vi "Shift Header to point to starting tag.vi"(6 "Byte stream offset\ninsertion point where \nnew data/tag added":u32, 7 "Litt/BigEnd":bool, 8 "error in":errorcluster, 9 "# bytes added\n(<0 means removed)":i32, 11 "Image Data":u8[](array[numeric])) -> (0 "error out":errorcluster, 1 "Shifted?":bool, 3 "Image Data Out":u8[](array[numeric]))   [LabVIEW 2013, in "Tiff reader.lvlib"]
doc: "This .vi shifts the data stream that is to be added into a stack so that the pointers now point to their new locations."
uses:
  Tiff reader.lvlib
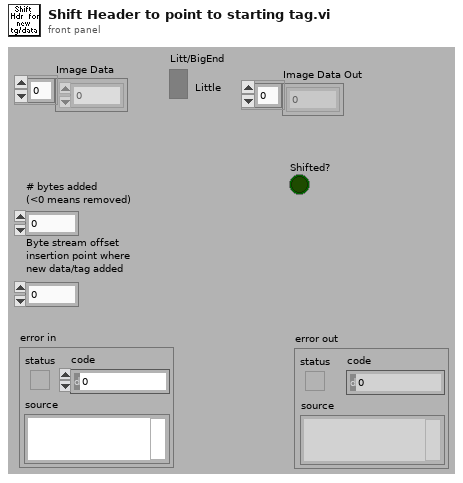
[diagram p1: front panel]
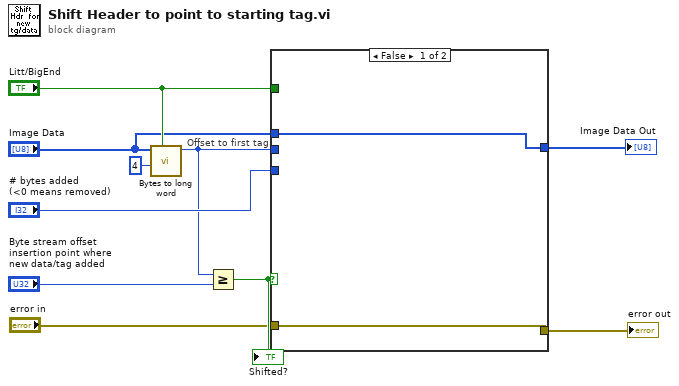
[diagram p0: block diagram]
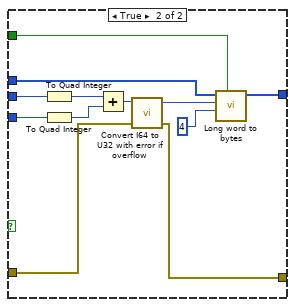
[diagram p2: hidden frame]
diagram:
  # "Offset to first tag"
  n1 = call "Bytes to long word.vi"("Litt/BigEnd"="Litt/BigEnd", "Index"=4, "Image Data in"="Image Data") -> ("U32"=w7:u32)  [unwired: 6 out]
  n2 = Greater Or Equal?(x=w7, y="Byte stream offset\ninsertion point where \nnew data/tag added") -> (x >= y?=w4:bool)
  "Shifted?" <- w4
  n3 = case shown="False" w4 {
    tunnel: "Image Data" -> [w12 w24]
    tunnel: [w12 w23] -> w6
    tunnel: w7 -> [_ w22]
    tunnel: "# bytes added\n(<0 means removed)" -> [_ w20]
    tunnel: "Litt/BigEnd" -> [_ w17]
    tunnel: "error in" -> [w11 w14]
    tunnel: [w11 w13] -> w2
    frame False {
    }
    frame True {
      n4 = To Quad Integer(1:w22) -> (0:w21:i64)
      n5 = To Quad Integer(1:w20) -> (0:w19:i64)
      n6 = Add(x=w21, y=w19) -> (x+y=w16:i64)
      n7 = call "Convert I64 to U32 with error if overflow.vi"("error in"=w14, "I64"=w16) -> ("error out"=w13:errorcluster, "U32"=w15:u32)  [unwired: 2 out]
      n8 = call "Long word to bytes.vi"("Litt/BigEnd"=w17, "Index"=4, "U32"=w15, "Image Data in"=w24) -> ("Image Data out"=w23:u8[])  [unwired: 5 out]
    }
  }
  "Image Data Out" <- w6
  "error out" <- w2
